vi "WSVCAP SHL Host LL SPI Build and Parse Write Message.vi"(0 "Write Data In [DUT Ordered]":u8[][](array[numeric]) format="%02x", 1 "Message In":string, 5 "Socket Mask [U16] In":u16=1 format="%04x", 7 "Cycle CMD Lengths (bits)":u8[](array[numeric]), 9 "Cycle CMD Delay (ticks)":u32[](array[numeric]), 11 "error in":errorcluster) -> (3 "Message Out":string, 4 "Write Data Out [DUT Ordered]":u8[][](array[numeric]) format="%02x", 6 "Socket Mask [U16] Out":u16=1 format="%04x", 8 "Cycle CMD Lengths Out (bits)":u8[](array[numeric]), 10 "Cycle CMD Delay Out (ticks)":u32[](array[numeric]), 15 "error out":errorcluster)   [LabVIEW 2012]
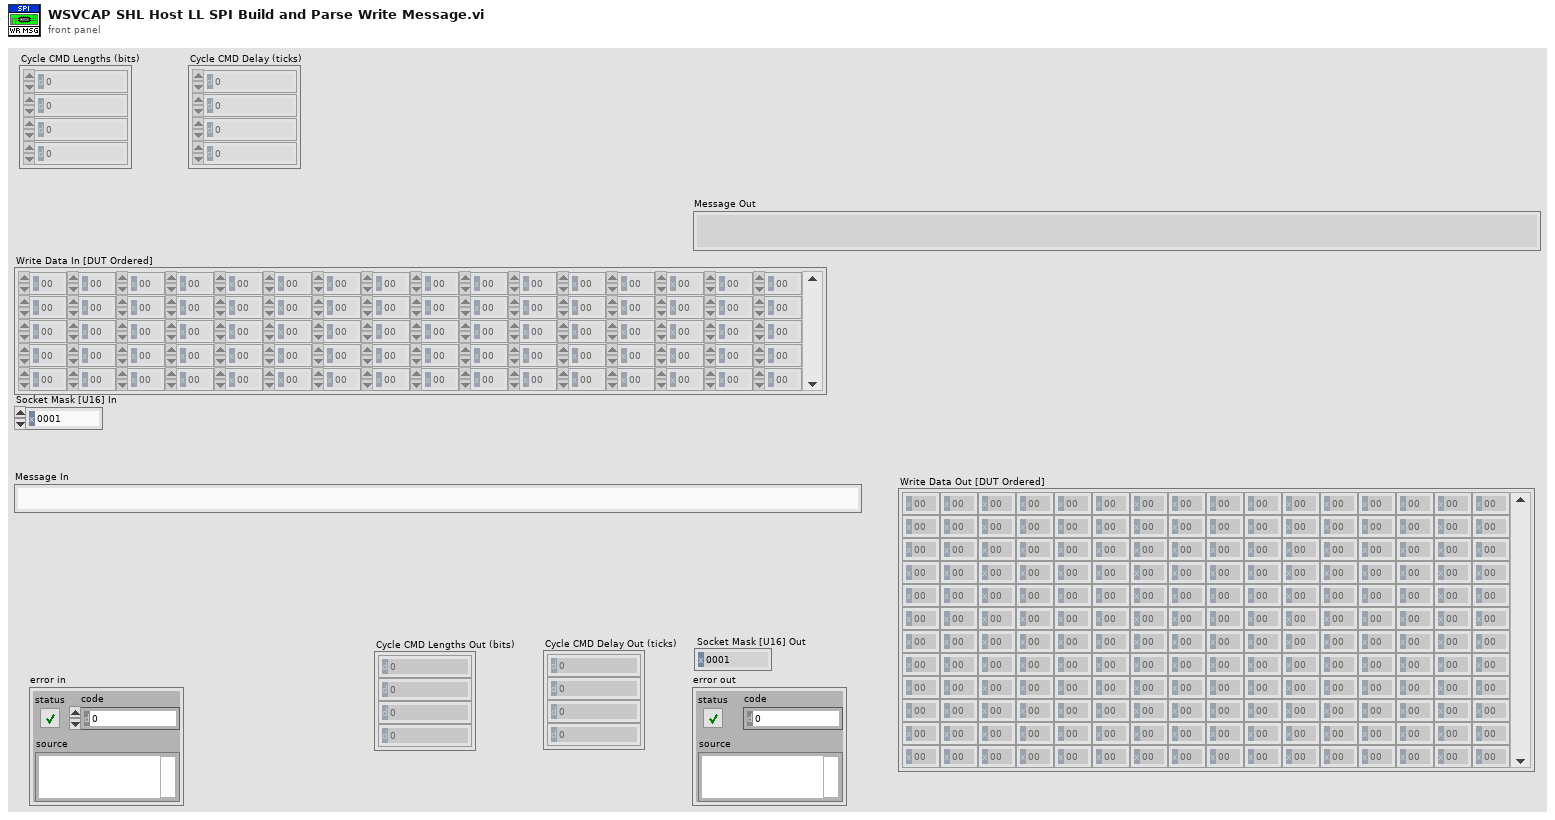
[diagram p1: front panel]
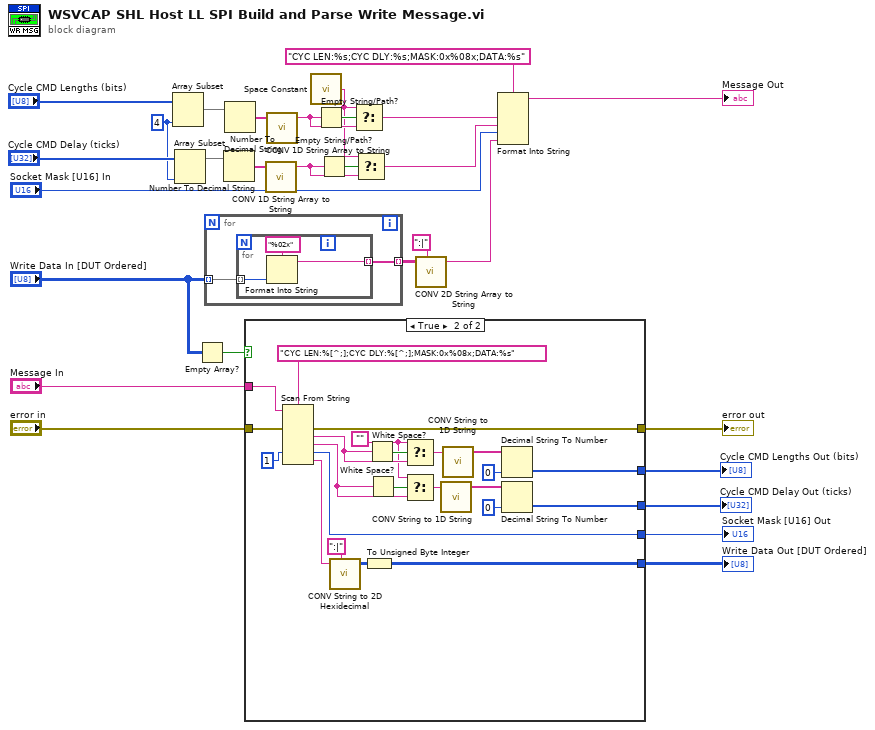
[diagram p0: block diagram]
diagram:
  w12 = 4 ("length")
  n1 = Array Subset(array="Cycle CMD Lengths (bits)", length=w12) -> (w15:u8[])  [unwired: 1 in]
  n2 = Array Subset(array="Cycle CMD Delay (ticks)", length=w12) -> (w13:u32[])  [unwired: 1 in]
  n3 = Empty Array?(array="Write Data In [DUT Ordered]") -> (empty?=w21:bool)
  n4 = for {
    tunnel: "Write Data In [DUT Ordered]" -> [w31] mode=indexing
    tunnel: [w30] -> w2 mode=indexing
    n5 = for {
      tunnel: w31 -> [w34] mode=indexing
      tunnel: [w33] -> w30 mode=indexing
      n6 = Format Into String(format string="%02x", w34) -> (resulting string=w33:string)  [unwired: 2 in, 1 out]
    }
  }
  n7 = Number To Decimal String(number=w13) -> (decimal integer string=w19:string[])  [unwired: 1 in]
  n8 = Number To Decimal String(number=w15) -> (decimal integer string=w20:string[])  [unwired: 1 in]
  n9 = case shown="True" w21 {
    tunnel: [_ w57] -> w27
    tunnel: [_ w55] -> w26
    tunnel: "error in" -> [w35 w53]
    tunnel: [w35 w52] -> w24
    tunnel: "Message In" -> [_ w50]
    tunnel: [_ w44] -> w18
    tunnel: [_ w43] -> w17
    frame False {
    }
    frame True {
      w36 = ""
      n10 = Scan From String(format string="CYC LEN:%[^;];CYC DLY:%[^;];MASK:0x%08x;DATA:%s", input string=w50, error in=w53, default 3=u16 1 ("Socket Mask [U16] Out")) -> (error out=w52:errorcluster, output 1=w39:string, output 2=w40:string, output 3=w55:u16, output 4=w54:string)  [unwired: 4 in, 2 out]
      n11 = call "CONV String to 2D Hexidecimal.vi"("String"=w54, "Delimiters (,;)"=":|") -> ("2-D Hexidecimal"=w58:u32[][])  [unwired: 7 in]
      n12 = To Unsigned Byte Integer(number=w58) -> (unsigned 8bit integer=w57:u8[][])
      n13 = White Space?(1:w39) -> (0:w38:bool)
      n14 = White Space?(1:w40) -> (0:w37:bool)
      n15 = Select(t=w36, s=w38, f=w39) -> (s? t:f=w42:string)
      n16 = Select(t=w36, s=w37, f=w40) -> (s? t:f=w41:string)
      n17 = call "CONV String to 1D String.vi"("String"=w41) -> ("1-D String"=w47:string[])  [unwired: 8 in]
      n18 = call "CONV String to 1D String.vi"("String"=w42) -> ("1-D String"=w48:string[])  [unwired: 8 in]
      n19 = Decimal String To Number(string=w48, default (0L)=u8 0 ("Read Data")) -> (number=w44:u8[])  [unwired: 1 in, 1 out]
      n20 = Decimal String To Number(string=w47, default (0L)=u64 0 ("Read Data")) -> (number=w43:u64[])  [unwired: 1 in, 1 out]
    }
  }
  "Write Data Out [DUT Ordered]" <- w27
  "Socket Mask [U16] Out" <- w26
  "error out" <- w24
  "Cycle CMD Lengths Out (bits)" <- w18
  "Cycle CMD Delay Out (ticks)" <- w17
  n21 = call "CONV 1D String Array to String.vi"("1-D String"=w19) -> ("String"=w8:string)  [unwired: 1 in, 7 out]
  n22 = call "CONV 1D String Array to String.vi"("1-D String"=w20) -> ("String"=w10:string)  [unwired: 1 in, 7 out]
  n23 = call <vilib>:"Space Constant.vi"() -> ("String"=w7:string)
  n24 = Empty String/Path?(string/path=w10) -> (empty?=w11:bool)
  n25 = Empty String/Path?(string/path=w8) -> (empty?=w9:bool)
  n26 = Select(t=w7, s=w11, f=w10) -> (s? t:f=w6:string)
  n27 = Select(t=w7, s=w9, f=w8) -> (s? t:f=w5:string)
  n28 = call "CONV 2D String Array to String.vi"("2-D String"=w2, "Delimiters (,;)"=":|") -> ("String"=w1:string)  [unwired: 7 in]
  n29 = Format Into String(format string="CYC LEN:%s;CYC DLY:%s;MASK:0x%08x;DATA:%s", w6, w5, "Socket Mask [U16] In", w1) -> (resulting string=→"Message Out":string)  [unwired: 2 in, 1 out]
